vi "Fetch Voltage Sweep.vi"(0 "VISA resource name":refnum<visa-resource-name>, 11 "error in (no error)":errorcluster) -> (4 "VISA resource name out":refnum<visa-resource-name>, 6 "Sweep Results":cluster{dbl[], dbl[]}(graph), 15 "error out":errorcluster)   [LabVIEW 2020, in "Keithley 648X Series.lvlib"]
doc: "Fetches the latest acquired set of voltage sweep readings.\n\n<B>Notes:</B> \n1)Use this VI only with other low-level VIs. The high-level VIs automatically incorporate this functionality. This VI does not check the instrument status. If you want to check the instrument status, call the <B>Error Query</B> VI at the conclusion of the sequence.\n2)<b>This VI is only valid for the model 6487 </b>"
uses:
  <instrlib>/Keithley 648X Series/Keithley 648X Series.lvlib
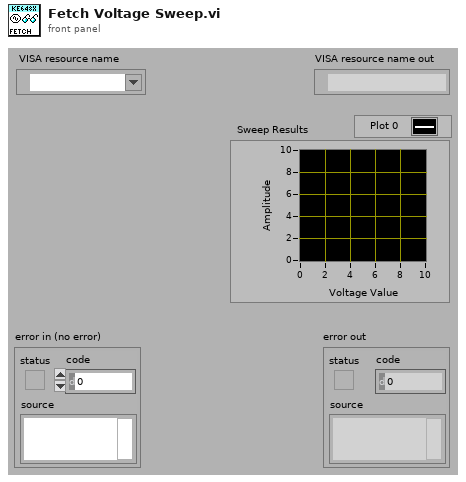
[diagram p1: front panel]
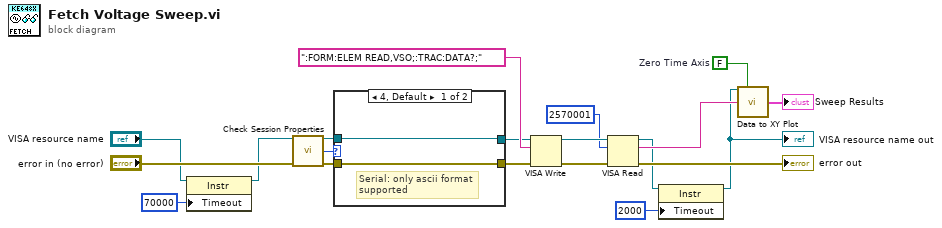
[diagram p0: block diagram]
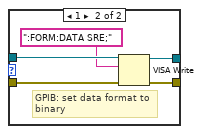
[diagram p2: hidden frame]
diagram:
  w8 = FALSE  # Zero Time Axis
  n1 = property class="Instr"(reference="VISA resource name", "Timeout"=u32 70000 ("General Settings:Timeout Value")) -> (reference out=w6:refnum<visa-resource-name>)  [unwired: 1 in, 1 out]
  n2 = call <instrlib>:"Check Session Properties.vi"("VISA resource name"=w6, "error in (no error)"="error in (no error)") -> ("VISA resource name out"=w14:refnum<visa-resource-name>, "Interface Type"=w15:u16, "error out"=w16:errorcluster)  [unwired: 10 in, 1 out]
  n3 = case shown="4, Default" w15 {
    tunnel: [w22 w27] -> w13
    tunnel: [w21 w26] -> w12
    tunnel: w16 -> [w21 w25]
    tunnel: w14 -> [w22 w24]
    frame 4, Default {
      # "Serial: only ascii format\nsupported"
    }
    frame 1 {
      # "GPIB: set data format to\nbinary"
      n4 = VISA Write(VISA resource name=w24, write buffer=":FORM:DATA SRE;", error in (no error)=w25) -> (VISA resource name out=w27:refnum<visa-resource-name>, error out=w26:errorcluster)  [unwired: 1 out]
    }
  }
  n5 = VISA Write(VISA resource name=w13, write buffer=":FORM:ELEM READ,VSO;:TRAC:DATA?;" ("Initiate"), error in (no error)=w12) -> (VISA resource name out=w19:refnum<visa-resource-name>, error out=w18:errorcluster)  [unwired: 1 out]
  n6 = VISA Read(VISA resource name=w19, byte count=u32 2570001, error in (no error)=w18) -> (VISA resource name out=w1:refnum<visa-resource-name>, read buffer=w9:string, error out=→"error out":errorcluster)  [unwired: 1 out]
  n7 = property class="Instr"(reference=w1, "Timeout"=u32 2000 ("General Settings:Timeout Value")) -> (reference out=w2:refnum<visa-resource-name>)  [unwired: 1 in, 1 out]
  "VISA resource name out" <- w2
  n8 = call <instrlib>:"Data to XY Plot.vi"("VISA resource name"=w2, "Zero Time Axis (T)"=w8, "String of Data"=w9) -> ("XY Graph"=→"Sweep Results":cluster{dbl[], dbl[]})  [unwired: 12 in]
